vi "Generator.vi"() -> ()   [LabVIEW 2022 SP3]
uses:
  <vilib>/DAQmx/read.llb/DAQmx Read (Analog DBL 1Chan 1Samp).vi
  d98ec7b3-635e-44d3-a42b-e01b1401c296.vi
  <vilib>/DAQmx/write.llb/DAQmx Write (Analog DBL 1Chan 1Samp).vi
  <vilib>/measure/matone.llb/Extract Single Tone Information 1 Chan.vi
  <vilib>/DAQmx/miscellaneous.llb/DAQmx Fill In Error Info.vi
  <vilib>/measure/NI_MABase.lvlib
  <vilib>/measure/NI_MAPro.lvlib
panel:
  in  "stop 3":bool
  in  "frequency 2":dbl=10.0 format="%0.2p"
  in  "signal type 2":T1(ring)
  in  "sampling info 2":cluster{"Fs":dbl, "#s":dbl}={"Fs"=1000.0, "#s"=1000.0} {"Fs" format="%.2p"}
  in  "square wave duty cycle (%) 2":dbl=50.0 format="%0.2f"
  in  "stop 2":bool
  out "Aquired":dbl(graph)
  out "size(s)":i32
  out "Generated":dbl[](graph)
  in  "frequency":dbl=10.0 format="%0.2p"
  in  "signal type":T1(ring)
  in  "sampling info":cluster{"Fs":dbl, "#s":dbl}={"Fs"=1000.0, "#s"=1000.0} {"Fs" format="%.2p"}
  in  "square wave duty cycle (%)":dbl=50.0 format="%0.2f"
  out "error constant":errorcluster
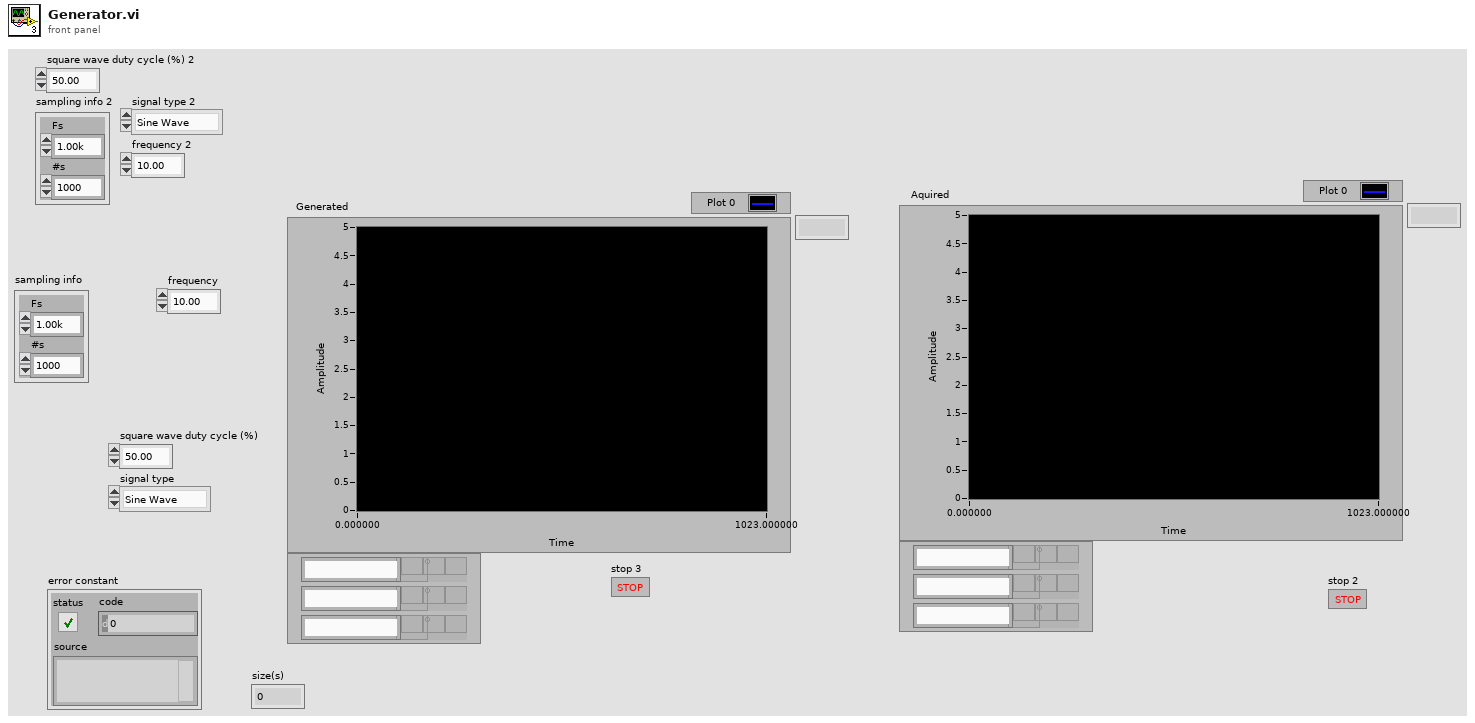
[diagram p1: front panel]
types:
  T1 = enum16{"Sine Wave", "Triangle Wave", "Square Wave", "Sawtooth Wave"}
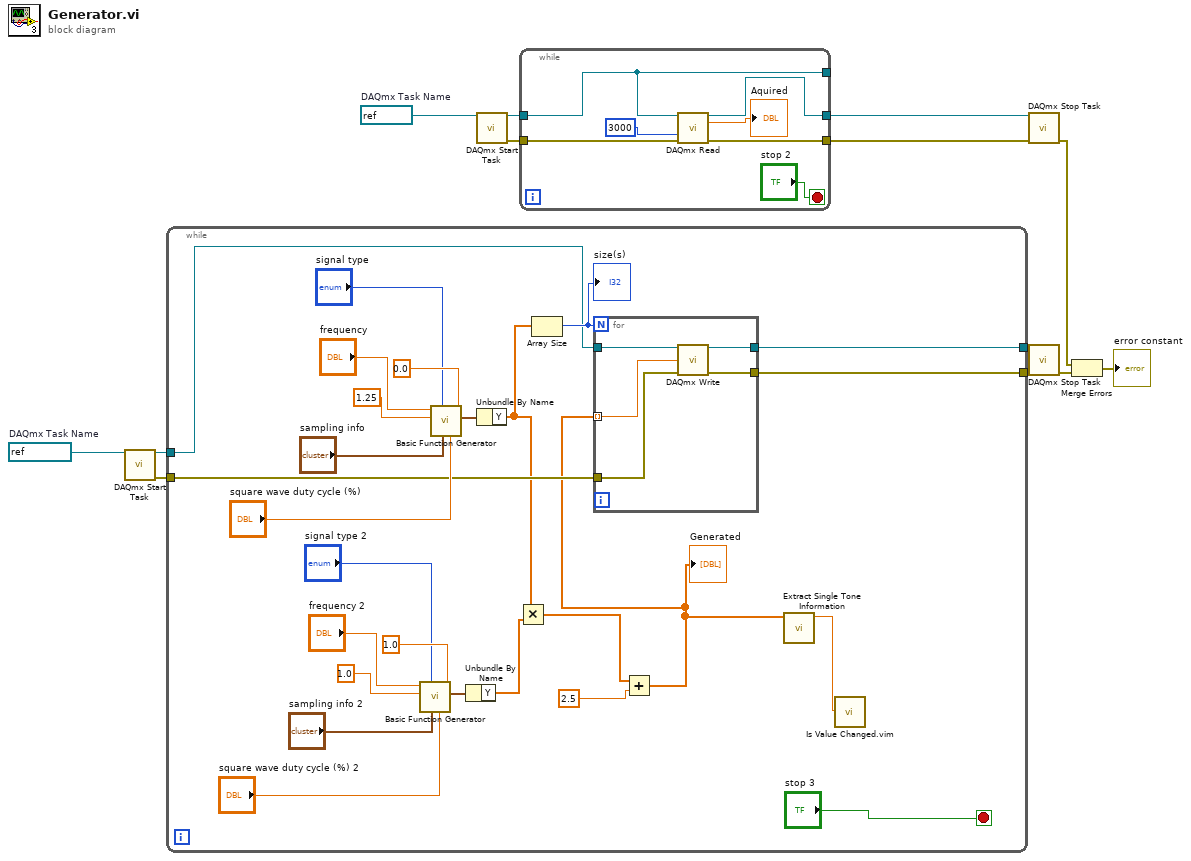
[diagram p0: block diagram]
diagram:
  w1 = refnum<k21> "V_IN"  # DAQmx Task Name
  w5 = refnum<k21> "V_OUT"  # DAQmx Task Name
  n1 = call <vilib>:"DAQmx Start Task.vi"("task/channels in"=w5) -> ("task out"=w13:refnum<k21>, "error out"=w12:errorcluster)  [unwired: 13 in]
  n2 = while {
    tunnel: w13 -> [w31]
    tunnel: w12 -> [w30]
    tunnel: [w29] -> w11
    tunnel: [w28] -> w10
    stop <- "stop 3" stop-if-true
    n3 = call <vilib>:"Basic Function Generator.vi"("offset"=1.0, "square wave duty cycle (%)"="square wave duty cycle (%) 2", "sampling info"="sampling info 2", "signal type"="signal type 2", "amplitude"=1.0, "frequency"="frequency 2") -> ("signal out"=w21:waveform(dbl))  [unwired: 3 in, 2 out]
    n4 = call <vilib>:"Basic Function Generator.vi"("offset"=0.0, "square wave duty cycle (%)"="square wave duty cycle (%)", "sampling info"="sampling info", "signal type"="signal type", "amplitude"=1.25, "frequency"="frequency") -> ("signal out"=w33:waveform(dbl))  [unwired: 3 in, 2 out]
    n5 = Unbundle By Name(w21) -> ("Y"=w20:dbl[])
    n6 = Unbundle By Name(w33) -> ("Y"=w19:dbl[])
    n7 = Multiply(x=w19, y=w20) -> (x*y=w17:dbl[])
    n8 = Array Size(array=w19) -> (size(s)=w32:i32)
    "size(s)" <- w32
    n9 = Add(x=w17, y=2.5) -> (x+y=w16:dbl[])
    "Generated" <- w16
    n10 = for {
      N: w32 -> [_]
      tunnel: w16 -> [w44] mode=indexing
      tunnel: w31 -> [w43]
      tunnel: w30 -> [w42]
      tunnel: [w41] -> w29
      tunnel: [w40] -> w28
      n11 = call-poly <vilib>:"DAQmx Write.vi"("task/channels in"=w43, "data"=w44, "error in"=w42) -> ("task out"=w41:refnum<k21>, "error out"=w40:errorcluster)  [unwired: 10 in, 1 out]
    }
    n12 = call-poly <vilib>:"Extract Single Tone Information.vi"("time signal in"=w16) -> ("detected frequency"=w15:dbl)  [unwired: 5 in, 5 out]
    n13 = call "Is Value Changed.vim"("value"=w15) -> ()  [unwired: 1 out]
  }
  n14 = call <vilib>:"DAQmx Start Task.vi"("task/channels in"=w1) -> ("task out"=w9:refnum<k21>, "error out"=w8:errorcluster)  [unwired: 13 in]
  n15 = while {
    tunnel: [w50] -> _
    tunnel: [w51] -> w6
    tunnel: w9 -> [w50]
    tunnel: w8 -> [w49]
    tunnel: [w45] -> w7
    stop <- "stop 2" stop-if-true
    n16 = call-poly <vilib>:"DAQmx Read.vi"("task/channels in"=w50, "timeout"=3000, "error in"=w49) -> ("task out"=w51:refnum<k21>, "data"=→"Aquired":dbl, "error out"=w45:errorcluster)  [unwired: 10 in]
  }
  n17 = call <vilib>:"DAQmx Stop Task.vi"("task/channels in"=w6, "error in"=w7) -> ("error out"=w4:errorcluster)  [unwired: 12 in, 1 out]
  n18 = call <vilib>:"DAQmx Stop Task.vi"("task/channels in"=w11, "error in"=w10) -> ("error out"=w3:errorcluster)  [unwired: 12 in, 1 out]
  n19 = Merge Errors(w4, w3) -> (→"error constant":errorcluster)
